vi "Change password FGV.vi"(8 "error in":errorcluster, 9 "Change Password in":bool, 11 "Enum":enum16{"Read", "Write"}(ring)) -> (0 "error Out":errorcluster, 1 "Change Password Out":bool)   [LabVIEW 2022 SP3]
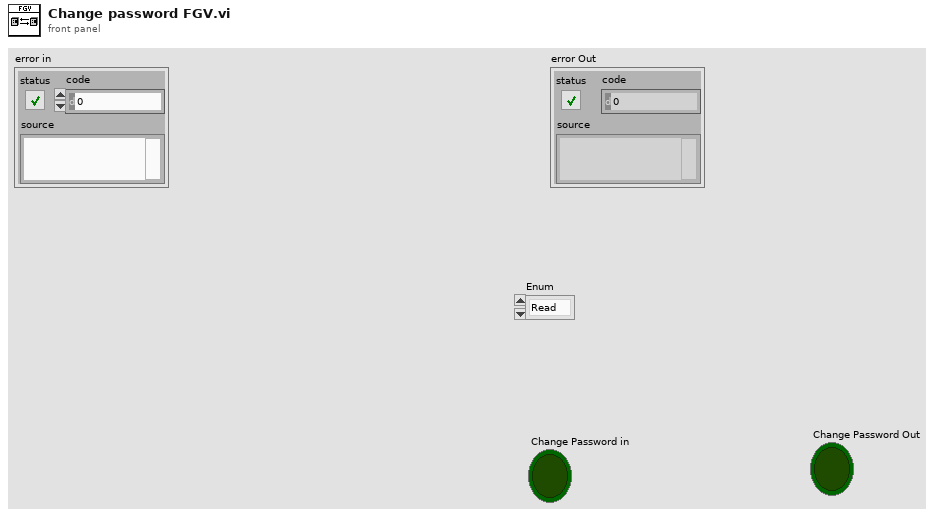
[diagram p1: front panel]
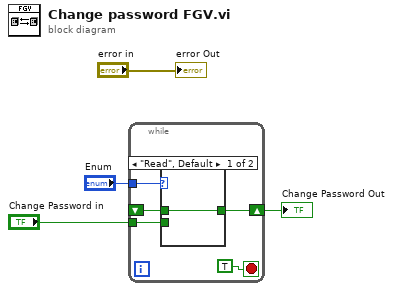
[diagram p0: block diagram]
diagram:
  n1 = while {
    tunnel: "Enum" -> [w9]
    tunnel: "Change Password in" -> [w7]
    shift-right: [w6] -> w2
    shift-left: _ -> [w5]
    stop <- TRUE stop-if-true
    n2 = case shown="\"Read\", Default" w9 {
      tunnel: w7 -> [_ w11]
      tunnel: [w10 w11] -> w6
      tunnel: w5 -> [w10 _]
      frame "Read", Default {
      }
      frame "Write" {
      }
    }
  }
  "Change Password Out" <- w2
  "error Out" <- "error in"
